vi "PH_O2_Watch.PC Write PSDB.vi"(0 "i ref in":refnum<vi>, 5 "error IO":errorcluster) -> (14 "i ref out":refnum<vi>, 19 "error out":errorcluster)   [LabVIEW 2014, in "PH_O2_Watch.lvlib"]
doc: "This is the proc case which writes data to the PHELIX shot data base."
uses:
  PH_O2_Watch.lvlib
  PH_Basics/PH_PSDBWriter/PH_PSDBWriter.lvlib
  PH_Basics/PH_StatusHandler/PH_StatusHandler.lvlib
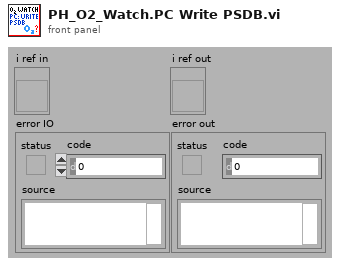
[diagram p1: front panel]
types:
  T1 = typedef "PH_O2_Watch.lvlib/PH_O2_Watch.i attribute.ctl" = cluster{"GUI Refs":cluster{"PreAlert":refnum<vi>, "Alert":refnum<vi>, "Failure":refnum<vi>, "Concentration":refnum<vi>, "Delete":refnum<vi>, "Limit":refnum<vi>}, "State PreAlert":T2, "State Alert":T2, "State Failure":T2, "Concentration":dbl, "Limit":dbl}
  T2 = typedef "PH_StatusHandler.lvlib/PH_StatusHandler.Status.ctl" = i16
  T3 = typedef "PH_PSDBWriter.lvlib/PH_PSDBWriter.Numeric dataset.ctl" = cluster{"name":string, "data":dbl, "unit":string}
  T4 = typedef "PH_PSDBWriter.lvlib/PH_PSDBWriter.String dataset.ctl" = cluster{"name":string, "data":string, "unit":string}
  T5 = typedef "PH_PSDBWriter.lvlib/PH_PSDBWriter.PSDB Dataset.ctl" = cluster{"Version":i32, "2D data Input":T6[], "Boolean Input":T8[], "Image Input":T9[], "Numeric Input":T3[], "String Input":T4[]}
  T6 = typedef "PH_PSDBWriter.lvlib/PH_PSDBWriter.2D dataset.ctl" = cluster{"name":string, "data":dbl[][], "axis description":T7}
  T7 = typedef "PSDB.lvlib/PSDB_AxisDescription.ctl" = cluster{"x axis label":string, "y axis label":string, "x axis unit":string, "y axis unit":string}
  T8 = typedef "PH_PSDBWriter.lvlib/PH_PSDBWriter.Boolean dataset.ctl" = cluster{"name":string, "data":bool, "unit":string}
  T9 = typedef "PH_PSDBWriter.lvlib/PH_PSDBWriter.Image dataset.ctl" = cluster{"name":string, "data":T10, "unit":string}
  T10 = typedef "IMAQ Image.ctl" = refnum<image>
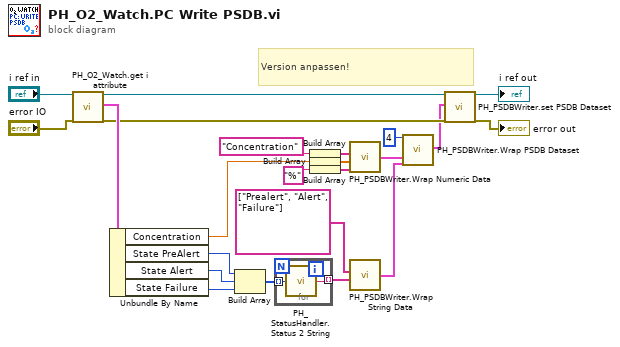
[diagram p0: block diagram]
diagram:
  # "Version anpassen!"
  n1 = call "PH_O2_Watch.get i attribute.vi"("i ref in"="i ref in", "error in (no error)"="error IO") -> ("i ref out"=w14:refnum<vi>, "i attribute"=w17:T1, "error out"=w16:errorcluster)  [unwired: 15 in]
  n2 = Unbundle By Name(w17) -> ("Concentration"=w9:dbl, "State PreAlert"=w18:T2, "State Alert"=w19:T2, "State Failure"=w20:T2)
  n3 = Build Array(w18, w19, w20) -> (w21:T2[])
  n4 = for {
    tunnel: w21 -> [w25] mode=indexing
    tunnel: [w24] -> w2 mode=indexing
    n5 = call "PH_StatusHandler.Status 2 String.vi"("Status"=w25) -> ("Status as string"=w24:string)
  }
  n6 = Build Array("Concentration" ("name")) -> (w4:string[])
  n7 = Build Array(w9) -> (w6:dbl[])
  n8 = Build Array("%" ("unit")) -> (w5:string[])
  n9 = call "PH_PSDBWriter.Wrap Numeric Data.vi"("Unit Array"=w5, "Data Array"=w6, "Name Array"=w4) -> ("PSDB Numeric Data Array"=w7:T3[])  [unwired: 1 in]
  n10 = call "PH_PSDBWriter.Wrap String Data.vi"("Data Array"=w2, "Name Array"=string[] ["Prealert", "Alert", "Failure"]) -> ("PSDB String Data Array"=w3:T4[])  [unwired: 2 in]
  n11 = call "PH_PSDBWriter.Wrap PSDB Dataset.vi"("Version"=4, "Numeric Input"=w7, "String Input"=w3) -> ("PSDB Dataset"=w12:T5)  [unwired: 16 in]
  n12 = call "PH_PSDBWriter.set PSDB Dataset.vi"("VI in"=w14, "PSDB Dataset"=w12, "error in (no error)"=w16) -> ("VI out"=→"i ref out":refnum<vi>, "error out"=→"error out":errorcluster)  [unwired: 15 in]
